vi "NewPower_Close.vi"(2 "error in":errorcluster, 3 "Language":T1, 4 "power485":refnum<visa-resource-name>="COM3") -> (0 "error out":errorcluster, 1 "Message":string)   [LabVIEW 2015]
uses:
  CustomControl/Lang_Control.ctl
  <vilib>/Instr/_visa.llb/VISA Configure Serial Port (Instr).vi
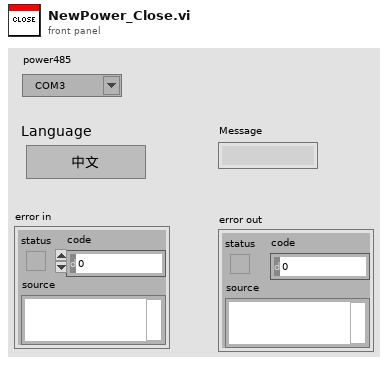
[diagram p1: front panel]
types:
  T1 = typedef "Lang_Control.ctl" = enum16{"中文", "English"}
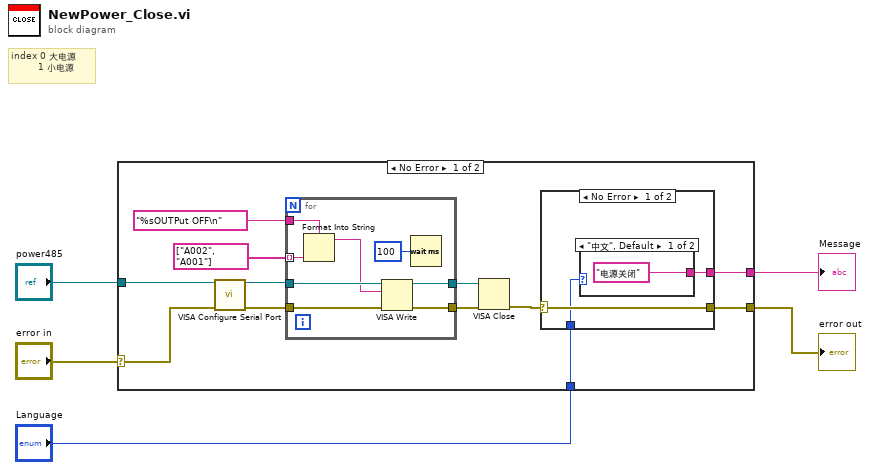
[diagram p0: block diagram]
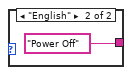
[diagram p2: hidden frame]
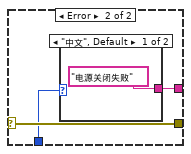
[diagram p3: hidden frame]
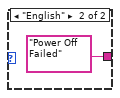
[diagram p4: hidden frame]
diagram:
  # "index 0 大电源\n         1 小电源"
  n1 = case shown="No Error" "error in" {
    selector: "error in" -> [w10 w36]
    tunnel: "power485" -> [w11 _]
    tunnel: [w9 w36] -> w4
    tunnel: "Language" -> [w8 _]
    tunnel: [w7 _] -> w1
    frame No Error {
      n2 = call-poly "VISA Configure Serial Port"("VISA resource name"=w11, "error in (no error)"=w10) -> ("VISA resource name out"=w12:refnum<visa-resource-name>, "error out"=w13:errorcluster)  [unwired: 12 in]
      n3 = for {
        tunnel: string[] ["A002", "A001"] -> [w35] mode=indexing
        tunnel: w13 -> [w33]
        tunnel: "%sOUTPut OFF\n" ("format string") -> [w30]
        tunnel: w12 -> [w34]
        tunnel: [w29] -> w15
        tunnel: [w32] -> w14
        n4 = Format Into String(format string=w30, w35) -> (resulting string=w31:string)  [unwired: 2 in, 1 out]
        n5 = VISA Write(VISA resource name=w34, write buffer=w31, error in (no error)=w33) -> (VISA resource name out=w29:refnum<visa-resource-name>, error out=w32:errorcluster)  [unwired: 1 out]
        n6 = Wait (ms)(milliseconds to wait=u32 100) -> ()  [unwired: 1 out]
      }
      n7 = VISA Close(VISA resource name=w15, error in (no error)=w14) -> (error out=w6:errorcluster)
      n8 = case shown="No Error" w6 {
        selector: w6 -> [w20 w25]
        tunnel: [w20 w25] -> w9
        tunnel: w8 -> [w19 w24]
        tunnel: [w18 w23] -> w7
        frame No Error {
          n9 = case shown="\"中文\", Default" w19 {
            tunnel: ["电源关闭" "Power Off"] -> w18
            frame "中文", Default {
            }
            frame "English" {
            }
          }
        }
        frame Error {
          n10 = case shown="\"中文\", Default" w24 {
            tunnel: ["电源关闭失败" "Power Off Failed"] -> w23
            frame "中文", Default {
            }
            frame "English" {
            }
          }
        }
      }
    }
    frame Error {
    }
  }
  "error out" <- w4
  "Message" <- w1
